vi "Voltage_reading.vi"(8 "error in (no error)":errorcluster {"code" format="%.0x"}, 10 "Combo Box":string(combo), 11 "resource string":string="USB0::0x2A8D::0x5001::MY58039196::INSTR") -> (0 "error out":errorcluster {"code" format="%.0x"}, 2 "Val":dbl[](array[numeric]) format="%.2p")   [LabVIEW 2021]
uses:
  <instrlib>/Keysight DAQ970/Keysight DAQ970.lvlib
panel:
  in  "ChannelList":string="110:118"
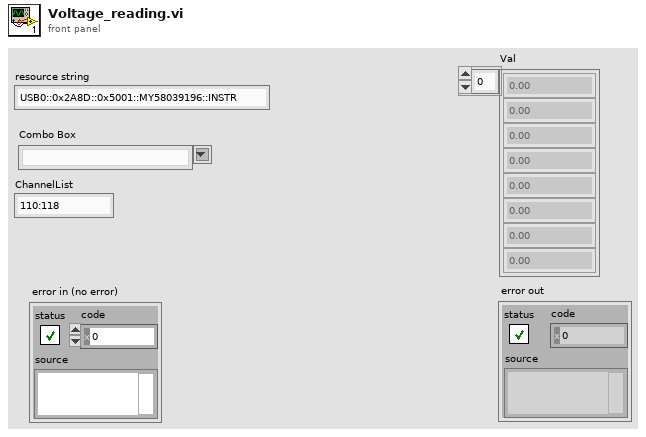
[diagram p1: front panel]
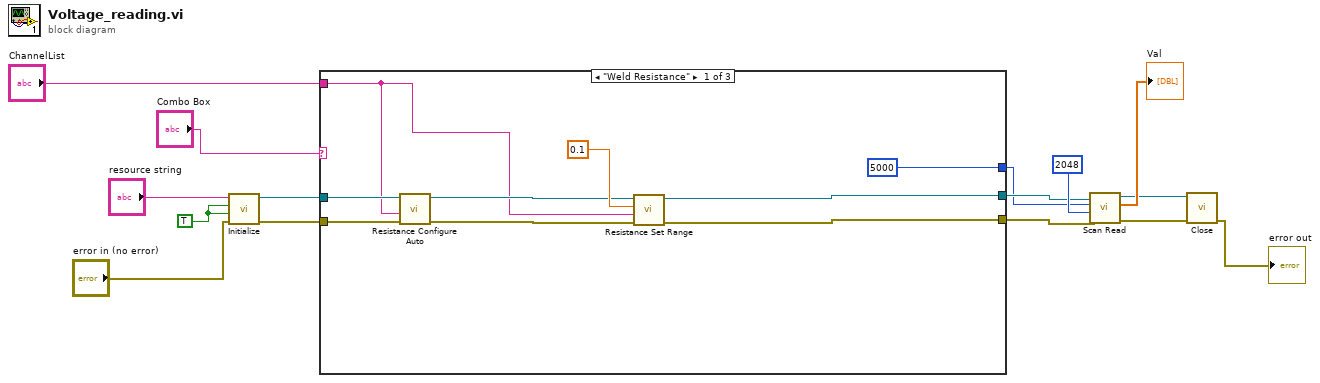
[diagram p0: block diagram]
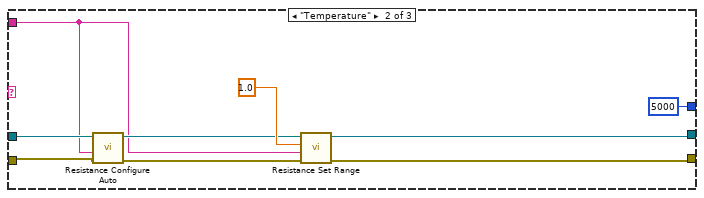
[diagram p2: hidden frame]
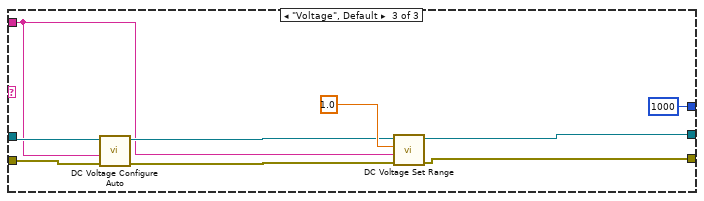
[diagram p3: hidden frame]
diagram:
  w8 = TRUE ("id query (Off)")
  n1 = call <instrlib>:"Initialize.vi"("error in (no error)"="error in (no error)", "reset device (Off)"=w8, "id query (Off)"=w8, "resource string"="resource string") -> ("error out"=w15:errorcluster, "instrument handle out"=w13:refnum<k15>)  [unwired: 6 in]
  n2 = case shown="\"Weld Resistance\"" "Combo Box" {
    tunnel: w13 -> [w18 w31 w39]
    tunnel: w15 -> [w17 w32 w40]
    tunnel: "ChannelList" -> [w16 w27 w37]
    tunnel: [w22 w25 w36] -> w7
    tunnel: [w23 w26 w35] -> w5
    tunnel: [5000 ("MaxTimeMilliseconds") 5000 ("MaxTimeMilliseconds") 1000 ("MaxTimeMilliseconds")] -> w1
    frame "Weld Resistance" {
      n3 = call <instrlib>:"Resistance Configure Auto.vi"("error in (no error)"=w17, "ChannelList"=w16, "instrument handle"=w18) -> ("error out"=w19:errorcluster, "instrument handle out"=w20:refnum<k15>)  [unwired: 7 in]
      n4 = call <instrlib>:"Resistance Set Range.vi"("error in (no error)"=w19, "ChannelList"=w16, "Range"=0.1, "instrument handle"=w20) -> ("error out"=w22:errorcluster, "instrument handle out"=w23:refnum<k15>)  [unwired: 6 in]
    }
    frame "Temperature" {
      n5 = call <instrlib>:"Resistance Configure Auto.vi"("error in (no error)"=w32, "ChannelList"=w27, "instrument handle"=w31) -> ("error out"=w28:errorcluster, "instrument handle out"=w29:refnum<k15>)  [unwired: 7 in]
      n6 = call <instrlib>:"Resistance Set Range.vi"("error in (no error)"=w28, "ChannelList"=w27, "Range"=1.0, "instrument handle"=w29) -> ("error out"=w25:errorcluster, "instrument handle out"=w26:refnum<k15>)  [unwired: 6 in]
    }
    frame "Voltage", Default {
      n7 = call <instrlib>:"DC Voltage Configure Auto.vi"("error in (no error)"=w40, "ChannelList"=w37, "instrument handle"=w39) -> ("error out"=w38:errorcluster, "instrument handle out"=w41:refnum<k15>)  [unwired: 7 in]
      n8 = call <instrlib>:"DC Voltage Set Range.vi"("error in (no error)"=w38, "ChannelList"=w37, "Range"=1.0, "instrument handle"=w41) -> ("error out"=w36:errorcluster, "instrument handle out"=w35:refnum<k15>)  [unwired: 6 in]
    }
  }
  n9 = call <instrlib>:"Scan Read.vi"("error in (no error)"=w7, "ValBufferSize"=2048, "MaxTimeMilliseconds"=w1, "instrument handle"=w5) -> ("error out"=w4:errorcluster, "Val"=→"Val":dbl[], "instrument handle out"=w2:refnum<k15>)  [unwired: 4 in, 1 out]
  n10 = call <instrlib>:"Close.vi"("error in (no error)"=w4, "instrument handle"=w2) -> ("error out"=→"error out":errorcluster)  [unwired: 9 in]
